vi "callConsoleUi.vi"(8 "error in (no error)":errorcluster, 11 "Handler.UserEvent.Console in":refnum<class "Handler.UserEvent.Console.lvclass">) -> (0 "error out":errorcluster, 3 "Handler.UserEvent.Console out":refnum<class "Handler.UserEvent.Console.lvclass">)   [LabVIEW 2017, in "Error Log.lvlib" / "Handler.UserEvent.Console.lvclass"]
uses:
  Handler.UserEvent.Console.lvclass
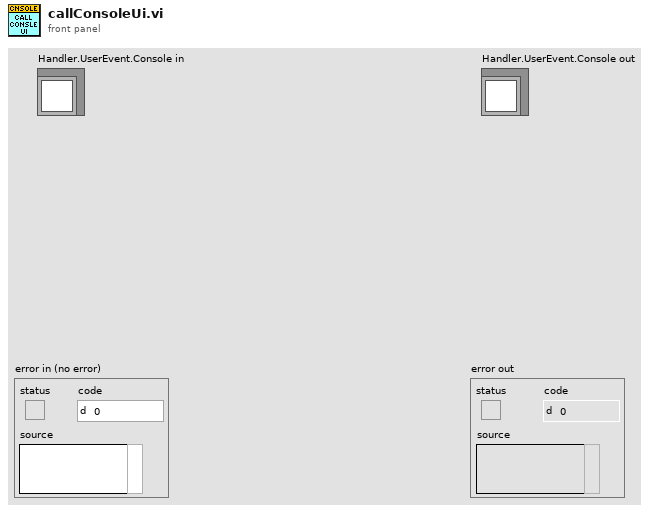
[diagram p1: front panel]
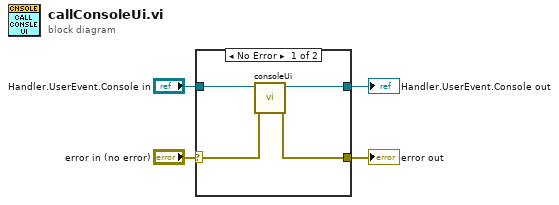
[diagram p0: block diagram]
diagram:
  n1 = case shown="No Error" "error in (no error)" {
    selector: "error in (no error)" -> [w6 w10]
    tunnel: [w5 w10] -> w3
    tunnel: [w7 w9] -> w1
    tunnel: "Handler.UserEvent.Console in" -> [w8 w9]
    frame No Error {
      n2 = call-dynamic "consoleUi.vi"("error in (no error)"=w6, "Handler.UserEvent.Console in"=w8) -> ("error out"=w5:errorcluster, "Handler.UserEvent.Console out"=w7:refnum<class "Handler.UserEvent.Console.lvclass">)  [unwired: 7 in, 1 out]
    }
    frame Error {
    }
  }
  "error out" <- w3
  "Handler.UserEvent.Console out" <- w1
